vi "Init.vi"(3 "Container State":T3, 4 "Previous State":variant, 5 "Previous Version":T2) -> (2 "Current State":T4={"Graph Visible Items"={"Plot Legend"=TRUE, "Scale Legend"=FALSE, "Graph Palette"=TRUE, "Cursor Legend"=FALSE, "X Scrollbar"=FALSE}, "View Table"=TRUE, "Table Visible Items"={"Vertical Scrollbar"=TRUE, "Horizontal Scrollbar"=TRUE, "Row Headers"=TRUE, "Column Headers"=TRUE, "Vertical Lines"=TRUE, "Horizontal Lines"=TRUE}, "Header Font"={"Font Name"="", "Size"=13, "Bold"=FALSE, "Italic"=FALSE, "Underline"=FALSE, "Strikeout"=FALSE, "Color"=0}, "Cell Font"={"Font Name"="", "Size"=13, "Bold"=FALSE, "Italic"=FALSE, "Underline"=FALSE, "Strikeout"=FALSE, "Color"=0}, "Description and Tip..."={"Description"="", "Tip"=""}, "Moveable Splitter Position"=420, "Measurement Cursor Configuration"={"relative to t0"={"enable relative time"=FALSE, "Relative times (DT)"=[], "color"=0}, "range"={"enable range"=FALSE, "T1"=0.025, "T2"=0.075, "Fixed interval (T2-T1)"=-1.0, "T1 color"=8404992, "T2 color"=8404992, "enable shading"=FALSE}, "periodic"={"enable periodic"=FALSE, "First event (E1)"=0.025, "Number events (Ei)"=2, "Event spacing (s)"=0.0, "First color"=16744512, "Events color"=16711680}, "absolute timestamp"={"enable absolute"=FALSE, "Timestamps (TS)"=[], "color"=2}}, "X Increment"=0.0, "X Scale"={"Label Visible"=FALSE, "Label Text"="", "Time Mode"=enum."Relative", "Format String"=""}, "Y Scale"={"Label Visible"=TRUE, "Label Text"="Time (s)", "Scaling"=enum."Engineering Units", "Format String"="%.2f"}, "Colors"={"background"=16777215, "major grid"=8355711, "minor grid"=12632256, "font"=0}, "Cursors"={"List"=[], "Tags"=[]}, "Plots"=[], "Plot Color Wheel"=[3381759, 32768, 982784, 4375295, 13827953, 13457919, 16757522, 4343295, 16728758, 12095254], "registered user events"=variant})   [LabVIEW 2017, in "Waveforms with Cursors.xctl"]
uses:
  <vilib>/addons/_XControls/Waveforms with Cursors/Waveforms with Cursors.xctl
  <vilib>/addons/_XControls/Waveforms with Cursors/Controls/State.ctl
  <vilib>/Utility/miscctls.llb/LVFontTypeDef.ctl
  <vilib>/addons/_XControls/Waveforms with Cursors/Controls/Waveform Cursor Configuration.ctl
  <vilib>/_xctls/Container State.ctl
  <vilib>/_xctls/Version.ctl
  <vilib>/_xctls/XControlSupport.lvlib
panel:
  in  "Tab Control":T1(tab)=enum."Default Control State"
  in  "Default Control State":T4={"Graph Visible Items"={"Plot Legend"=FALSE, "Scale Legend"=FALSE, "Graph Palette"=TRUE, "Cursor Legend"=FALSE, "X Scrollbar"=FALSE}, "View Table"=TRUE, "Table Visible Items"={"Vertical Scrollbar"=TRUE, "Horizontal Scrollbar"=TRUE, "Row Headers"=TRUE, "Column Headers"=TRUE, "Vertical Lines"=TRUE, "Horizontal Lines"=TRUE}, "Header Font"={"Font Name"="", "Size"=15, "Bold"=FALSE, "Italic"=FALSE, "Underline"=FALSE, "Strikeout"=FALSE, "Color"=0}, "Cell Font"={"Font Name"="", "Size"=15, "Bold"=FALSE, "Italic"=FALSE, "Underline"=FALSE, "Strikeout"=FALSE, "Color"=0}, "Description and Tip..."={"Description"="", "Tip"=""}, "Moveable Splitter Position"=420, "Measurement Cursor Configuration"={"relative to t0"={"enable relative time"=FALSE, "Relative times (DT)"=[], "color"=0}, "range"={"enable range"=FALSE, "T1"=0.025, "T2"=0.075, "Fixed interval (T2-T1)"=-1.0, "T1 color"=8404992, "T2 color"=8404992, "enable shading"=FALSE}, "periodic"={"enable periodic"=FALSE, "First event (E1)"=0.025, "Number events (Ei)"=2, "Event spacing (s)"=0.0, "First color"=16744512, "Events color"=16711680}, "absolute timestamp"={"enable absolute"=FALSE, "Timestamps (TS)"=[], "color"=2}}, "X Increment"=0.0, "X Scale"={"Label Visible"=TRUE, "Label Text"="Time (s)", "Time Mode"=enum."Relative", "Format String"="%_4g"}, "Y Scale"={"Label Visible"=TRUE, "Label Text"="Engineering Units", "Scaling"=enum."Engineering Units", "Format String"="%.2f"}, "Colors"={"background"=16777215, "major grid"=8355711, "minor grid"=12632256, "font"=0}, "Cursors"={"List"=[], "Tags"=[]}, "Plots"=[], "Plot Color Wheel"=[3381759, 32768, 982784, 4375295, 13827953, 13457919, 16757522, 4343295, 16728758, 12095254], "registered user events"=variant}
  in  "Default Indicator State":T4={"Graph Visible Items"={"Plot Legend"=FALSE, "Scale Legend"=FALSE, "Graph Palette"=TRUE, "Cursor Legend"=FALSE, "X Scrollbar"=FALSE}, "View Table"=TRUE, "Table Visible Items"={"Vertical Scrollbar"=TRUE, "Horizontal Scrollbar"=TRUE, "Row Headers"=TRUE, "Column Headers"=TRUE, "Vertical Lines"=TRUE, "Horizontal Lines"=TRUE}, "Header Font"={"Font Name"="", "Size"=15, "Bold"=FALSE, "Italic"=FALSE, "Underline"=FALSE, "Strikeout"=FALSE, "Color"=0}, "Cell Font"={"Font Name"="", "Size"=15, "Bold"=FALSE, "Italic"=FALSE, "Underline"=FALSE, "Strikeout"=FALSE, "Color"=0}, "Description and Tip..."={"Description"="", "Tip"=""}, "Moveable Splitter Position"=420, "Measurement Cursor Configuration"={"relative to t0"={"enable relative time"=FALSE, "Relative times (DT)"=[], "color"=0}, "range"={"enable range"=FALSE, "T1"=0.025, "T2"=0.075, "Fixed interval (T2-T1)"=-1.0, "T1 color"=8404992, "T2 color"=8404992, "enable shading"=FALSE}, "periodic"={"enable periodic"=FALSE, "First event (E1)"=0.025, "Number events (Ei)"=2, "Event spacing (s)"=0.0, "First color"=16744512, "Events color"=16711680}, "absolute timestamp"={"enable absolute"=FALSE, "Timestamps (TS)"=[], "color"=2}}, "X Increment"=0.0, "X Scale"={"Label Visible"=TRUE, "Label Text"="Time (s)", "Time Mode"=enum."Relative", "Format String"="%_4g"}, "Y Scale"={"Label Visible"=TRUE, "Label Text"="Engineering Units", "Scaling"=enum."Engineering Units", "Format String"="%.2f"}, "Colors"={"background"=16777215, "major grid"=8355711, "minor grid"=12632256, "font"=0}, "Cursors"={"List"=[], "Tags"=[]}, "Plots"=[], "Plot Color Wheel"=[3381759, 32768, 982784, 4375295, 13827953, 13457919, 16757522, 4343295, 16728758, 12095254], "registered user events"=variant}
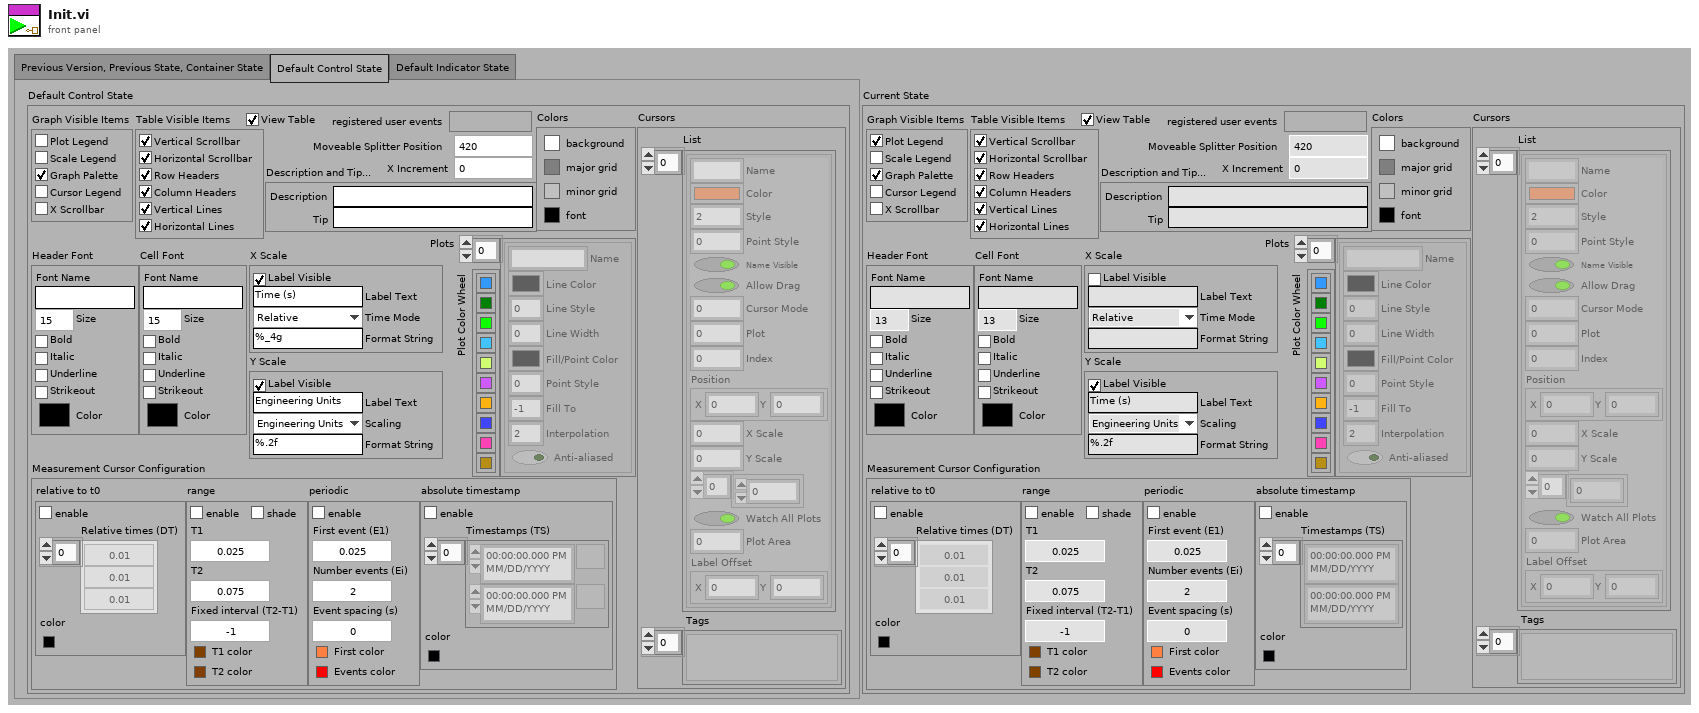
[diagram p1: front panel]
types:
  T1 = enum32{"Previous Version, Previous State, Container State", "Default Control State", "Default Indicator State"}
  T2 = typedef "XControlSupport.lvlib/Version.ctl" = cluster{"Major":u16, "Minor":u16, "Fix":u16, "Build":u16}
  T3 = typedef "XControlSupport.lvlib/Container State.ctl" = cluster{"Indicator?":bool, "Run Mode?":bool, " Refnum":refnum<vi>}
  T4 = typedef "Waveforms with Cursors.xctl/State.ctl" = cluster{"Graph Visible Items":cluster{"Plot Legend":bool, "Scale Legend":bool, "Graph Palette":bool, "Cursor Legend":bool, "X Scrollbar":bool}, "View Table":bool, "Table Visible Items":cluster{"Vertical Scrollbar":bool, "Horizontal Scrollbar":bool, "Row Headers":bool, "Column Headers":bool, "Vertical Lines":bool, "Horizontal Lines":bool}, "Header Font":T5, "Cell Font":T5, "Description and Tip...":cluster{"Description":string, "Tip":string}, "Moveable Splitter Position":i32, "Measurement Cursor Configuration":T6, "X Increment":dbl, "X Scale":cluster{"Label Visible":bool, "Label Text":string, "Time Mode":enum16{"Relative", "Absolute"}, "Format String":string}, "Y Scale":cluster{"Label Visible":bool, "Label Text":string, "Scaling":enum16{"Engineering Units", "Voltage"}, "Format String":string}, "Colors":cluster{"background":u32, "major grid":u32, "minor grid":u32, "font":u32}, "Cursors":cluster{"List":cluster{"Name":string, "Color":u32, "Style":i32, "Point Style":u8, "Name Visible":bool, "Allow Drag":bool, "Cursor Mode":u32, "Plot":i32, "Index":i32, "Position":cluster{"X":dbl, "Y":dbl}, "X Scale":u32, "Y Scale":u32, "Watch Plots":i32[], "Watch All Plots":bool, "Plot Area":i32, "Label Offset":cluster{"X":dbl, "Y":dbl}}[], "Tags":variant[]}, "Plots":cluster{"Name":string, "Line Color":u32, "Line Style":u8, "Line Width":u8, "Fill/Point Color":u32, "Point Style":u8, "Fill To":i16, "Interpolation":u8, "Anti-aliased":bool}[], "Plot Color Wheel":u32[], "registered user events":variant}
  T5 = typedef "LVFontTypeDef.ctl" = cluster{"Font Name":string, "Size":u16, "Bold":bool, "Italic":bool, "Underline":bool, "Strikeout":bool, "Color":u32}
  T6 = typedef "Waveforms with Cursors.xctl/Waveform Cursor Configuration.ctl" = cluster{"relative to t0":cluster{"enable relative time":bool, "Relative times (DT)":dbl[], "color":u32}, "range":cluster{"enable range":bool, "T1":dbl, "T2":dbl, "Fixed interval (T2-T1)":dbl, "T1 color":u32, "T2 color":u32, "enable shading":bool}, "periodic":cluster{"enable periodic":bool, "First event (E1)":dbl, "Number events (Ei)":i32, "Event spacing (s)":dbl, "First color":u32, "Events color":u32}, "absolute timestamp":cluster{"enable absolute":bool, "Timestamps (TS)":timestamp[], "color":u32}}
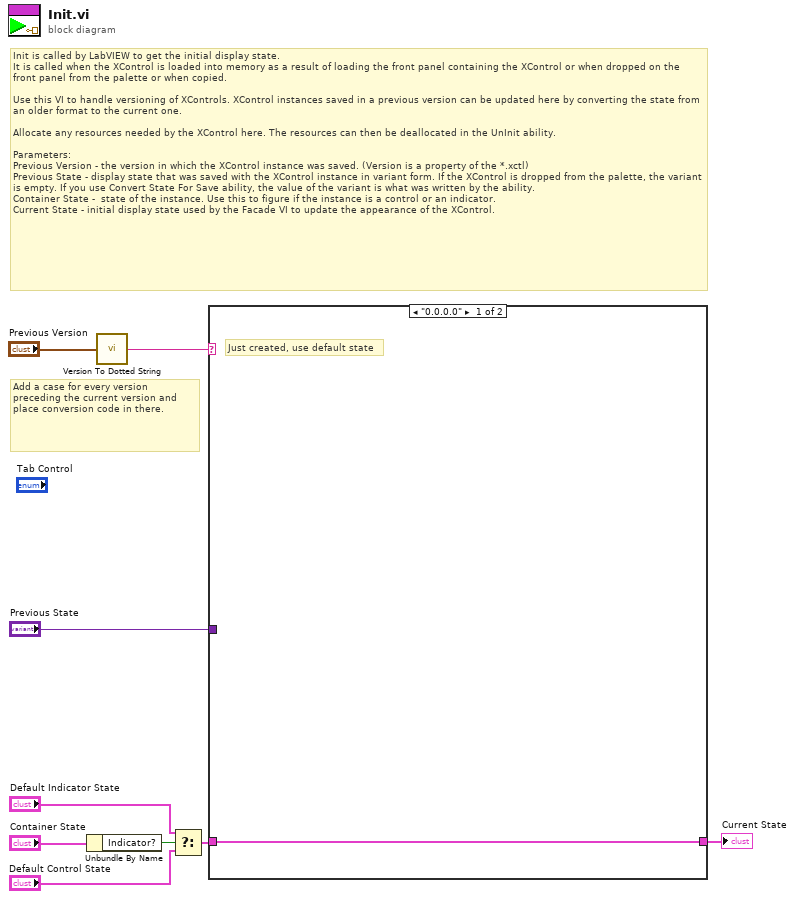
[diagram p0: block diagram]
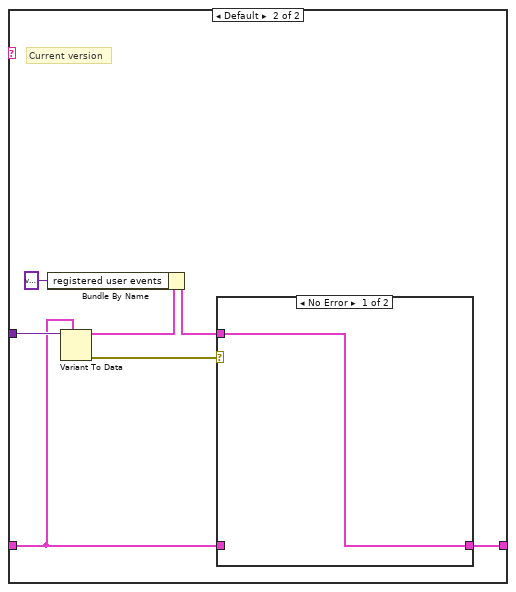
[diagram p2: hidden frame]
diagram:
  # "Add a case for every version preceding the current version and place conversion code in there."
  # "Init is called by LabVIEW to get the initial display state.\nIt is called when the XControl is loaded into memory as a result of loading the front panel containing the XControl or when dropped on the front panel from the palette or when copied.\n\nUse this VI to handle versioning of XControls. XControl instances saved in a previous version can be updated here by converting the state from an older format to the current one.\n\nAllocate any resources needed by the XControl here. The resources can then be deallocated in the UnInit ability.\n\nParameters:\nPrevious Version - the version in which the XControl instance was saved. (Version is a property of the *.xctl)\nPrevious State - display state that was saved with the XControl instance in variant form. If the XControl is dropped from the palette, the variant is empty. If you use Convert State For Save ability, the value of the variant is what was written by the ability. \nContainer State -  state of the instance. Use this to figure if the instance is a control or an indicator.\nCurrent State - initial display state used by the Facade VI to update the appearance of the XControl."
  n1 = Unbundle By Name("Container State") -> ("Indicator?"=w4:bool)
  n2 = call <vilib>:"Version To Dotted String.vi"("Version"="Previous Version") -> ("String Version"=w1:string)
  n3 = Select(t="Default Indicator State", s=w4, f="Default Control State") -> (s? t:f=w3:T4)
  n4 = case shown="\"0.0.0.0\"" w1 {
    tunnel: "Previous State" -> [_ w17]
    tunnel: [w10 w15] -> w8
    tunnel: w3 -> [w10 w14]
    frame "0.0.0.0" {
      # "Just created, use default state"
    }
    frame Default {
      # "Current version"
      n5 = Variant To Data(type=w14, Variant=w17) -> (data=w13:T4, error out=w16:errorcluster)  [unwired: 1 in]
      n6 = Bundle By Name(cluster=w13, "registered user events"=variant) -> (w11:T4)
      n7 = case shown="No Error" w16 {
        tunnel: w11 -> [w18 _]
        tunnel: [w18 w19] -> w15
        tunnel: w14 -> [_ w19]
        frame No Error {
        }
        frame Error {
          # "Error converting previously \nsaved state. Use default instead."
        }
      }
    }
  }
  "Current State" <- w8
